vi "Thorlabs_TDC001.constructor.vi"(0 "name":string, 2 "data in":string, 5 "error in (no error)":errorcluster) -> (14 "i ref out":refnum<vi>, 16 "data out":string, 19 "error out":errorcluster)   [LabVIEW 2014, in "Thorlabs_TDC001.lvlib"]
doc: "This is the constructor of a class.\n\nLicense Agreement for this software:\n\nCopyright (C)\nGesellschaft für Schwerionenforschung, GSI\nPlanckstr. 1\n64291 Darmstadt\nGermany\n\nContact: D.Beck@gsi.de \n\nThis program is free software; you can redistribute it and/or modify it under the terms of the \nGNU General Public License as published by the Free Software Foundation; either version 2 of \nthe license, or (at your option) any later version.\n\nThis program is distributed in the hope that it will be useful, but WITHOUT ANY WARRANTY; \nwithout even the implied warranty of MERCHANTABILITY or FITNESS FOR A PARTICULAR PURPOSE. See the GNU General License for more details (http://www.gnu.org).\n\nGesellschaft für Schwerionenforschung, GSI\nPlanckstr. 1, 64291 Darmstadt, Germany\nFor all questions and ideas contact: M.Richter@gsi.de, H.Brand@gsi.de or D.Beck@gsi.de.\nLast update: 16-JUN-2004"
uses:
  Thorlabs_TDC001.lvlib
  CS_Core/CSApplicationBaseClasses/DeviceBase/DeviceBase.myEventNames.ctl
  CS_Core/CSApplicationBaseClasses/DeviceBase/DeviceBase.lvlib
  CS_Core/CSSystem/CSSystemLib/CSSystemLib.lvlib
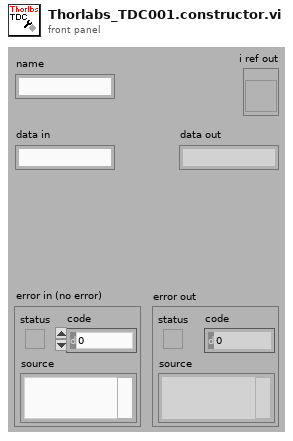
[diagram p1: front panel]
types:
  T1 = enum16{"SetAttribute", "GetAttribute", "CreateAttribute", "DestroyAttribute", "DestroyAllAtributes"}
  T2 = typedef "DeviceBase.lvlib/DeviceBase.myEventNames.ctl" = enum16{"lvmsg://Initialize", "lvmsg://Close", "lvmsg://Configure", "lvmsg://Reset", "lvmsg://IDQuery"}
  T3 = typedef "Thorlabs_TDC001.lvlib/Thorlabs_TDC001.i attribute.ctl" = cluster{"SerialNo":i32, "ChannelID":i32}
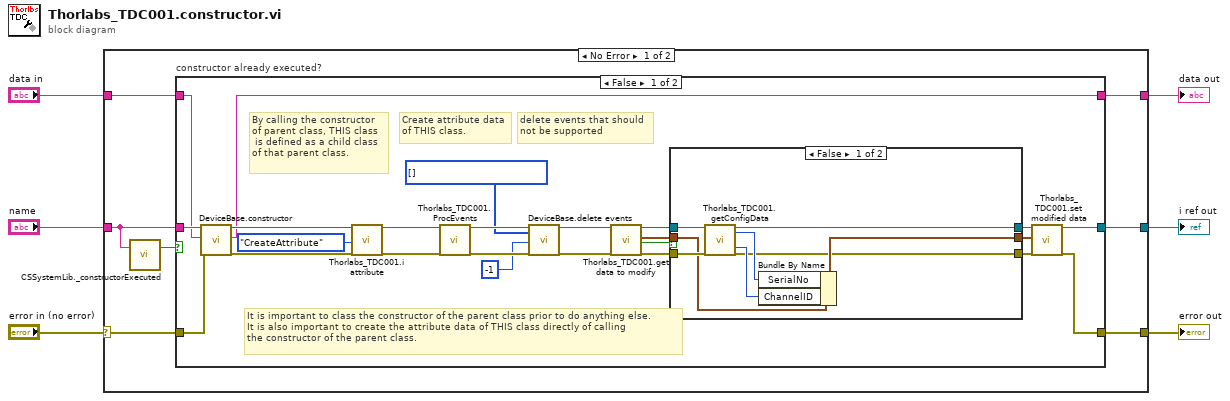
[diagram p0: block diagram]
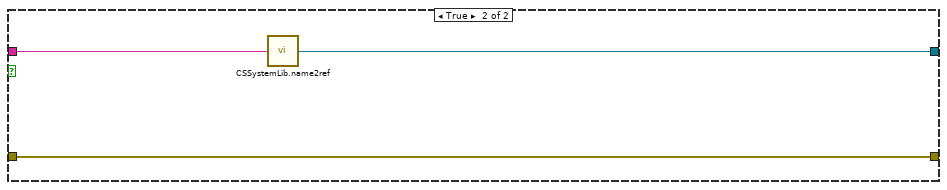
[diagram p3: hidden frame]
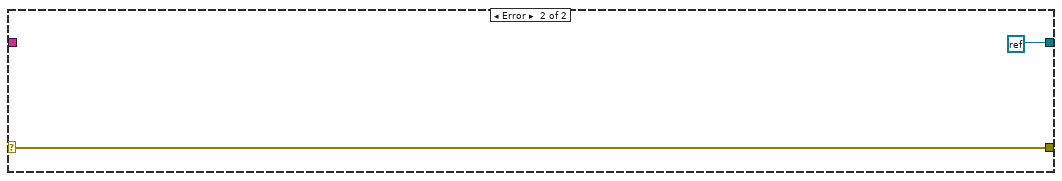
[diagram p4: hidden frame]
diagram:
  n1 = case shown="No Error" "error in (no error)" {
    selector: "error in (no error)" -> [w11 w52]
    tunnel: "name" -> [w10 _]
    tunnel: [w13 refnum<k0> refnum ("Not a Refnum Constant")] -> w5
    tunnel: [w12 w52] -> w4
    tunnel: "data in" -> [w8 _]
    tunnel: [w7 _] -> w1
    frame No Error {
      n2 = call "CSSystemLib._constructorExecuted.vi"("name"=w10) -> ("constructor executed?"=w9:bool)  [unwired: 18 in]
      n3 = case "constructor already executed?" shown="False" w9 {
        tunnel: w10 -> [w34 w51]
        tunnel: [w21 w50] -> w13
        tunnel: [w20 w49] -> w12
        tunnel: w11 -> [w31 w49]
        tunnel: w8 -> [w30 _]
        tunnel: [w25 _] -> w7
        frame False {
          w27 = T2[] [] items=["lvmsg://Initialize", "lvmsg://Close", "lvmsg://Configure", "lvmsg://Reset", "lvmsg://IDQuery"] ("events")
          # "delete events that should\nnot be supported"
          # "It is important to class the constructor of the parent class prior to do anything else.\nIt is also important to create the attribute data of THIS class directly of calling\nthe constructor of the parent class."
          # "Create attribute data\nof THIS class."
          # "By calling the constructor\nof parent class, THIS class\n is defined as a child class\nof that parent class."
          n4 = call "DeviceBase.constructor.vi"("name"=w34, "data in"=w30, "error in (no error)"=w31) -> ("i ref out"=w37:refnum<vi>, "data out"=w25:string, "error out"=w36:errorcluster)  [unwired: 14 in]
          n5 = call "Thorlabs_TDC001.i attribute.vi"("VI Refnum"=w37, "Action"=T1."CreateAttribute", "error in (no error)"=w36) -> ("VI Refnum out"=w33:refnum<vi>, "error out"=w32:errorcluster)  [unwired: 14 in, 1 out]
          n6 = call "Thorlabs_TDC001.ProcEvents.vi"("i ref in"=w33, "error in (no error)"=w32) -> ("i ref out"=w29:refnum<vi>, "error out"=w28:errorcluster)  [unwired: 16 in]
          n7 = call "DeviceBase.delete events.vi"("i ref in"=w29, "events"=w27, "ms timeout (10000)"=-1, "error in (no error)"=w28) -> ("i ref out"=w24:refnum<vi>, "error out"=w23:errorcluster)  [unwired: 13 in, 1 out]
          n8 = call "Thorlabs_TDC001.get data to modify.vi"("i ref in"=w24, "error in (no error)"=w23) -> ("i ref out"=w19:refnum<vi>, "i attribute"=w15:T3, "timed out"=w22:bool, "error out"=w17:errorcluster)  [unwired: 14 in]
          n9 = case shown="False" w22 {
            tunnel: w19 -> [w45 w48]
            tunnel: [w43 w48] -> w18
            tunnel: w17 -> [w44 w47]
            tunnel: [w38 w47] -> w16
            tunnel: w15 -> [w42 w46]
            tunnel: [w40 w46] -> w14
            frame False {
              n10 = call "Thorlabs_TDC001.getConfigData.vi"("i ref in"=w45, "error in (no error)"=w44) -> ("i ref out"=w43:refnum<vi>, "SerialNo"=w39:i32, "ChannelID"=w41:i32, "error out"=w38:errorcluster)  [unwired: 14 in]
              n11 = Bundle By Name(cluster=w42, "SerialNo"=w39, "ChannelID"=w41) -> (w40:T3)
            }
            frame True {
            }
          }
          n12 = call "Thorlabs_TDC001.set modified data.vi"("i ref in"=w18, "i attribute"=w14, "error in (no error)"=w16) -> ("i ref out"=w21:refnum<vi>, "error out"=w20:errorcluster)  [unwired: 15 in]
        }
        frame True {
          n13 = call "CSSystemLib.name2ref.vi"("name"=w51) -> ("obj refnum"=w50:refnum<vi>)
        }
      }
    }
    frame Error {
    }
  }
  "i ref out" <- w5
  "error out" <- w4
  "data out" <- w1
